vi "UHR-Fleezers Control (host) - Lorentz v4.vi"() -> ()   [LabVIEW 2014] (continued)
    n3458 = call-poly <vilib>:"Mean.vi"("X"=w4753) -> ("mean"=w4652:dbl)  [unwired: 1 out]
    "T2 X" <- w4652
    n3459 = Subtract(x=w4607, y=w4748) -> (x-y=w4747:dbl[])
    n3460 = Add(1:w4577, 2:w4581) -> (0:w4580:waveform(dbl))  [unwired: 1 in, 1 out]
    n3461 = Square(x=w4747) -> (x^2=w4746:dbl[])
    n3462 = Divide(x=w4580, y=2.0) -> (x/y=w4578:waveform(dbl))
    n3463 = Negate(x=w4753) -> (-x=w4619:dbl[])
    n3464 = call-poly <vilib>:"Mean.vi"("X"=w4746) -> ("mean"=w4745:dbl)  [unwired: 1 out]
    n3465 = Negate(x=w4652) -> (-x=w4651:dbl)
    n3466 = Square Root(x=w4745) -> (sqrt(x)=w4744:dbl)
    n3467 = Add(x=w4650, y=w4619) -> (x+y=w4754:dbl[])
    n3468 = Add(x=w4653, y=w4651) -> (x+y=w4772:dbl)
    n3469 = Multiply(x=10.0, y=w4744) -> (x*y=→"RMS (Ang)":dbl)
    n3470 = Divide(x=w4754, y=2.0) -> (x/y=w4622:dbl[])
    n3471 = Subtract(x=w4653, y=w4651) -> (x-y=→"Difference":dbl)
    n3472 = Build Array(w4581, w4577, w4578) -> (→"Force":waveform(dbl)[])
    n3473 = Select(t=w4619, s="Only check fixed trap T2", f=w4622) -> (s? t:f=→"Vec Mean of T1 T2":dbl[])
    n3474 = Divide(x=w4772, y=2.0) -> (x/y=w4563:dbl)
    "Mean" <- w4563
    n3475 = feedback-in #17("Trap Trig. Fl.") -> ()
    n3476 = feedback #17("Trap Trig. Fl.") -> (w4669:bool)
    n3477 = And(x=w4671, y=w4669) -> (x .and. y?=w4670:bool)
    n3478 = case "If have just turned off triggering" shown="True" w4670 {
      tunnel: w4574 -> [_ w4998]
      tunnel: w4665 -> [_ w4997]
      frame False {
      }
      frame True {
        w4996 = FALSE ("FPGA Trap Trig")
        n3479 = xnode "Read/Write Control"("FPGA VI Reference In"=w4998, "error in"=w4997, "FPGA Trap Trig"=w4996) -> ("FPGA VI Reference Out"=w4995:T50, "error out"=w4994:errorcluster)
        n3480 = xnode "Read/Write Control"("FPGA VI Reference In"=w4995, "error in"=w4994, "TTrig?"=w4996) -> ()  [unwired: 2 out]
        n3481 = local write "Initializing"(FALSE ("Initializing")) -> ()
        n3482 = local write "Triggered"(FALSE ("Triggered")) -> ()
        n3483 = local write "Waiting"(FALSE ("Waiting")) -> ()
      }
    }
    n3484 = Not(x=w4669) -> (.not. x?=w4682:bool)
    n3485 = And(x="Trap Trig. Fl.", y=w4682) -> (x .and. y?=w4679:bool)
    n3486 = Or(x=w4679, y="Reinitialize") -> (x .or. y?=w4668:bool)
    n3487 = feedback #18(w4675) -> (w4680:string)
    n3488 = Select(t=w4675, s=w4679, f=w4680) -> (s? t:f=w4674:string)
    n3489 = Select(t=w4675, s="Reinitialize", f=w4674) -> (s? t:f=w4673:string)
    n3490 = local read "Tether"() -> (w4756:bool)
    n3491 = feedback #19(0) -> (w4677:i32)
    n3492 = case "For determining if there is a tether still" shown="True" w4756 {
      tunnel: w4563 -> [_ w5107]
      frame False {
      }
      frame True {
        n3493 = Greater?(x="Lost Tether Alarm Threshold (pN)", y=w5107) -> (0:w5105:bool)
        n3494 = case shown="True" w5105 {
          frame False {
          }
          frame True {
            w5108 = FALSE ("Value (Signaling)")
            n3495 = flat-sequence {
              frame #0 {
                # "stop only if saving"
                n3496 = local read "Saving..."() -> (w5120:bool)
                n3497 = And(x=w5120, y="TA Cancel Save?") -> (x .and. y?=w5119:bool)
                n3498 = local write "Stop Saving"(w5119) -> ()
              }
              frame #1 {
                n3499 = case shown="True" "TA Green Off?" {
                  frame False {
                  }
                  frame True {
                    w5123 = FALSE ("Fl. Triggered...")
                    n3500 = local write "Fl. Triggered..."(w5123) -> ()
                    n3501 = property on="Green Laser ON" class="Bool (strict)"("Val(Sgnl)"=w5123) -> ()  [unwired: 2 in, 2 out]
                  }
                }
              }
            }
            n3502 = local read "Time tether formed"() -> (w5114:timestamp)
            n3503 = Get Date/Time In Seconds() -> (seconds since 1Jan1904=w5115:timestamp)
            n3504 = Subtract(x=w5115, y=w5114) -> (x-y=w5113:dbl)
            n3505 = Number To Decimal String(number=w5113) -> (decimal integer string=w5110:string)  [unwired: 1 out]
            n3506 = local read "Messages"() -> (w5117:string)
            n3507 = call <vilib>:"Beep.vi"() -> ()  [unwired: 3 in, 9 out]
            n3508 = Concatenate Strings("Lost tether (" ("Message to add"), w5110, " s)." ("string")) -> (w5112:string)
            n3509 = local write "Tether"(FALSE ("Tether")) -> ()
            n3510 = call "Update messages.vi"("Message to add"=w5112, "Old message string"=w5117) -> ("New message string"=w5116:string)
            n3511 = local write "Messages"(w5116) -> ()
            n3512 = property on="Fl. Triggered..." class="Bool (strict)"("Val(Sgnl)"=w5108) -> ()  [unwired: 2 in, 2 out]
            n3513 = local write "Dip for Protein"(w5108) -> ()
            n3514 = property on="Trap Pos. FB ON" class="Bool (strict)"("Val(Sgnl)"=w5108) -> ()  [unwired: 2 in, 2 out]
            n3515 = property on="Trap Trig. Fl." class="Bool (strict)"("Val(Sgnl)"=w5108) -> ()  [unwired: 2 in, 2 out]
          }
        }
      }
    }
    n3516 = case "For triggering actions based on the trap position (e.g., turning the excitation laser on if trap under feedback moves so far)" shown="True" "Trap Trig. Fl." {
      tunnel: w4479 -> [_ w5011]
      tunnel: w4673 -> [_ w5010]
      tunnel: ["" ("t") w5009] -> w4681
      tunnel: w4668 -> [_ w5008]
      tunnel: [0 ("t") w5007] -> w4678
      tunnel: w4677 -> [_ w5006]
      tunnel: w4574 -> [_ w5005]
      tunnel: w4665 -> [_ w5004]
      frame False {
      }
      frame True {
        n3517 = case shown="\"Wait for trigger\"" w5010 {
          tunnel: w5011 -> [w5028 _ _ w5076]
          tunnel: [w5025 w5057 "" ("t") w5079] -> w5009
          tunnel: w5008 -> [_ _ _ w5067]
          tunnel: [w5024 w5054 0 ("t") w5068] -> w5007
          tunnel: w5006 -> [_ w5056 _ w5074]
          tunnel: w5005 -> [w5013 w5051 _ w5070]
          tunnel: w5004 -> [w5012 w5050 _ w5069]
          frame "Wait for trigger" {
            n3518 = local read "Trap Trig. (FPGA)"() -> (w5016:bool)
            n3519 = Subtract(x=w5028, y="Mean T1 Position\nto compare (nm)") -> (x-y=w5021:dbl[])
            n3520 = call <vilib>:"Std Deviation and Variance.vi"("X"=w5021) -> ("mean"=→"mean":dbl, "standard deviation"=→"standard\ndeviation":dbl)  [unwired: 1 in, 1 out]
            n3521 = Array Max & Min(array=w5021) -> (max value=→"max value":dbl, min value=→"min value":dbl)  [unwired: 2 out]
            n3522 = Greater?(x=w5021, y="Threshold (nm)") -> (0:w5031:bool[])
            n3523 = case shown="True" w5016 {
              tunnel: w5013 -> [_ w5037]
              tunnel: w5012 -> [_ w5036]
              tunnel: [FALSE ("TTrig?") w5035] -> w5019
              frame False {
              }
              frame True {
                n3524 = xnode "Read/Write Control"("FPGA VI Reference In"=w5037, "error in"=w5036) -> ("TTrig?"=w5035:bool)  [unwired: 2 out]
              }
            }
            n3525 = Or Array Elements(Boolean array=w5031) -> (logical OR=w5018:bool)
            n3526 = Select(t=w5019, s=w5016, f=w5018) -> (s? t:f=w5017:bool)
            n3527 = Not(x=w5016) -> (.not. x?=w5015:bool)
            n3528 = And(x=w5017, y=w5015) -> (x .and. y?=w5014:bool)
            n3529 = Select(t="Triggered", s=w5017, f="Wait for trigger") -> (s? t:f=w5025:string)
            n3530 = case shown="True" w5017 {
              tunnel: [0 0] -> w5024
              tunnel: w5013 -> [_ w5042]
              tunnel: w5012 -> [_ w5041]
              frame False {
                "Waiting" <- TRUE ("Waiting")
              }
              frame True {
                n3531 = xnode "Read/Write Control"("FPGA VI Reference In"=w5042, "error in"=w5041, "TTrig?"=FALSE) -> ()  [unwired: 2 out]
                n3532 = local read "Messages"() -> (w5045:string)
                n3533 = call <vilib>:"Beep.vi"() -> ()  [unwired: 12 in]
                n3534 = call "Update messages.vi"("Message to add"="Unwinding trigger.", "Old message string"=w5045) -> ("New message string"=w5046:string)
                n3535 = local write "Messages"(w5046) -> ()
                n3536 = local write "Waiting"(FALSE ("Waiting")) -> ()
                "Triggered" <- TRUE ("Triggered")
              }
            }
            n3537 = case "Only need to turn on laser if host triggered" shown="True" w5014 {
              frame False {
              }
              frame True {
                n3538 = property on="Green Laser ON" class="Bool (strict)"("Val(Sgnl)"=TRUE ("Value (Signaling)")) -> ()  [unwired: 2 in, 2 out]
              }
            }
          }
          frame "Triggered" {
            n3539 = local read "Trap Trig. (FPGA)"() -> (w5053:bool)
            n3540 = Increment(x=w5056) -> (x+1=w5054:i32)
            n3541 = Greater Or Equal?(x=w5054, y="Fl. ON time (n)") -> (x >= y?=w5052:bool)
            n3542 = Select(t="Wait for trigger", s=w5052, f="Triggered" ("t")) -> (s? t:f=w5057:string)
            n3543 = And(x=w5052, y=w5053) -> (x .and. y?=w5049:bool)
            n3544 = case shown="True" w5049 {
              tunnel: w5051 -> [_ w5061]
              tunnel: w5050 -> [_ w5060]
              frame False {
              }
              frame True {
                n3545 = xnode "Read/Write Control"("FPGA VI Reference In"=w5061, "error in"=w5060, "FPGA Trap Trig"=TRUE) -> ()  [unwired: 2 out]
              }
            }
            n3546 = case shown="True" w5052 {
              frame False {
              }
              frame True {
                w5063 = FALSE ("Value (Signaling)")
                n3547 = local write "Triggered"(w5063) -> ()
                n3548 = local write "Waiting"(TRUE ("Waiting")) -> ()
                n3549 = property on="Green Laser ON" class="Bool (strict)"("Val(Sgnl)"=w5063) -> ()  [unwired: 2 in, 2 out]
              }
            }
          }
          frame "Do nothing" {
          }
          frame "Initialize", Default {
            n3550 = Increment(x=w5074) -> (x+1=w5078:i32)
            n3551 = Select(t=1, s=w5067, f=w5078) -> (s? t:f=w5068:i32)
            n3552 = feedback #20(w5076) -> (w5082:dbl[])
            n3553 = Build Array (concatenate)(w5076, w5082) -> (w5075:dbl[])
            n3554 = Greater Or Equal?(x=w5068, y="Wait to get offset (n)") -> (x >= y?=w5071:bool)
            n3555 = Select(t=w5076, s=w5067, f=w5075) -> (s? t:f=w5077:dbl[])
            n3556 = feedback-in #20(w5077) -> ()
            n3557 = call-poly <vilib>:"Mean.vi"("X"=w5077) -> ("mean"=w5072:dbl)  [unwired: 1 out]
            n3558 = local write "Mean T1 Position\nto compare (nm)"(w5072) -> ()
            n3559 = case shown="True" w5067 {
              tunnel: w5070 -> [_ w5088]
              tunnel: w5069 -> [_ w5087]
              frame False {
              }
              frame True {
                w5084 = FALSE ("FPGA Trap Trig")
                n3560 = xnode "Read/Write Control"("FPGA VI Reference In"=w5088, "error in"=w5087, "FPGA Trap Trig"=w5084) -> ("FPGA VI Reference Out"=w5086:T50, "error out"=w5085:errorcluster)
                n3561 = xnode "Read/Write Control"("FPGA VI Reference In"=w5086, "error in"=w5085, "TTrig?"=w5084) -> ()  [unwired: 2 out]
              }
            }
            n3562 = Select(t="Wait for trigger", s=w5071, f="Initialize") -> (s? t:f=w5079:string)
            n3563 = case shown="True" w5071 {
              tunnel: w5072 -> [_ w5091]
              tunnel: w5070 -> [_ w5100]
              tunnel: w5069 -> [_ w5099]
              frame False {
                n3564 = local write "Waiting"(FALSE ("Waiting")) -> ()
                "Initializing" <- TRUE ("Initializing")
              }
              frame True {
                n3565 = local read "Threshold (nm)"() -> (w5103:dbl)
                n3566 = local read "AOM X Cal (nm/MHz)"() -> (w5102:dbl)
                n3567 = Add(x=w5091, y=w5103) -> (x+y=w5104:dbl)
                n3568 = Divide(x=w5104, y=w5102) -> (x/y=w5101:dbl)
                n3569 = call "IR AOM freq to word.vi"("Frequency In (MHz)"=w5101) -> ("Frequency Word Out (double)"=w5098:dbl)
                n3570 = local write "Initializing"(FALSE ("Initializing")) -> ()
                n3571 = local write "Waiting"(TRUE ("Waiting")) -> ()
                n3572 = To Quad Integer(1:w5098) -> (0:w5097:i64)
                n3573 = xnode "Read/Write Control"("FPGA VI Reference In"=w5100, "error in"=w5099, "FPGA TTrig Thresh"=w5097) -> ("FPGA VI Reference Out"=w5094:T50, "error out"=w5093:errorcluster)
                n3574 = xnode "Read/Write Control"("FPGA VI Reference In"=w5094, "error in"=w5093, "FPGA Trap Trig"=TRUE) -> ()  [unwired: 2 out]
              }
            }
          }
        }
      }
    }
    n3575 = feedback-in #18(w4681) -> ()
    n3576 = feedback-in #19(w4678) -> ()
    n3577 = xnode ("Read/Write Control")("FPGA VI Reference In"=w4473, "error in"=w4764) -> ("FPGA VI Reference Out"=w4565:T50, "error out"=w4666:errorcluster, "AI2 Y Sum Set 1"=w4813:i16, "AI2 Y Sum Set 2"=w4812:i16, "AI1 X Set 1"=w4704:fxp<+/-,16,1>, "AI1 X Set 2"=w4703:fxp<+/-,16,1>, "Trap Pos FB Int Signal"=→"Trap Pos FB Int Signal":fxp<+/-,24,9>, "Trap Pos FB Int-Norm Signal"=→"Trap Pos FB Int-Norm Signal":fxp<+/-,16,1>, "Trap Pos FB Action"=w4697:i64, "Scanning"=→"AOD Scanning":bool, "Scan I"=→"AOD Scan I":u64, "Scanning MCL"=w4815:bool, "Scan I (MCL)"=→"MCL Scan I":u64, "Green FB Sum"=w4777:i16, "Trap Pos FB Action"=w4664:i64, "TTrig Fin Thresh"=w4660:i64, "Red FB Intensity"=w4647:i16, "Blue Intensity"=w4642:i16, "BD1 Frequency Out 1"=w4582:u64)
    "MCL Scanning" <- w4815
    "Trap Pos FB Action" <- w4697
    n3578 = Divide(x=w4647, y=3276.7) -> (x/y=w4646:dbl)
    "Red laser intensity (V)" <- w4646
    n3579 = Divide(x=w4642, y=3276.7) -> (x/y=w4641:dbl)
    "Blue laser intensity (V)" <- w4641
    n3580 = Divide(x=w4777, y=3276.7) -> (x/y=w4645:dbl)
    "Green laser intensity (V)" <- w4645
    n3581 = local read "FB Trig Integrate"() -> (w4658:u32)
    n3582 = Divide(x=w4664, y=w4658) -> (x/y=w4657:dbl)
    "TTrig Sig (Int)" <- w4657
    n3583 = Bundle(w4645, w4646, w4641) -> (→"Fluorescence laser intensities plot":cluster{dbl, dbl, dbl})  [unwired: 1 in]
    n3584 = Divide(x=w4660, y=w4658) -> (x/y=w4655:dbl)
    "TTrig Fin Thresh (Int)" <- w4655
    n3585 = local read "AOM X Cal (nm/MHz)"() -> (w4663:dbl)
    n3586 = local read "AI2 (V)"() -> (w4814:cluster{"Set 1":dbl, "Set 2":dbl})
    n3587 = Bundle By Name(cluster=w4814, "Set 1"=w4813, "Set 2"=w4812) -> (w4584:cluster{"Set 1":dbl, "Set 2":dbl})
    n3588 = Divide(x=w4697, y=327.67) -> (x/y=→"Action (%)":dbl)
    n3589 = case shown="True" "Semi Passive Mode" {
      tunnel: w4563 -> [_ w4881]
      frame False {
      }
      frame True {
        n3590 = local read "Target Force (pN)"() -> (w4879:dbl)
        n3591 = Less?(x="Jump Force (pN)", y=w4879) -> (x < y?=w4877:bool)
        n3592 = case shown="False" w4877 {
          tunnel: "Jump Force (pN)" -> [w4887 w4890]
          tunnel: w4881 -> [w4886 w4889]
          tunnel: [w4885 w4888] -> w4880
          frame False {
            n3593 = Less?(x=w4887, y=w4886) -> (x < y?=w4885:bool)
          }
          frame True {
            n3594 = Greater?(x=w4890, y=w4889) -> (0:w4888:bool)
          }
        }
        n3595 = case shown="False" w4880 {
          frame False {
            n3596 = local read "Trap Pos. FB ON"() -> (w4882:bool)
            n3597 = case shown="False" w4882 {
              frame False {
              }
              frame True {
                n3598 = property on="Trap Pos. FB ON" class="Bool (strict)"("Val(Sgnl)"=FALSE) -> ()  [unwired: 2 in, 2 out]
              }
            }
          }
          frame True {
            n3599 = property on="Trap Pos. FB ON" class="Bool (strict)"("Val(Sgnl)"=TRUE) -> ()  [unwired: 2 in, 2 out]
          }
        }
      }
    }
    n3600 = local read "Trap X (AI1)"() -> (w4717:T15)
    n3601 = call "IR AOM word double to freq.vi"("Frequency Word In (double)"=w4655) -> ("Frequency Out (MHz)"=w4654:dbl)
    n3602 = call "IR AOM word double to freq.vi"("Frequency Word In (double)"=w4657) -> ("Frequency Out (MHz)"=w4656:dbl)
    n3603 = Divide(x=w4584, y=3276.7) -> (x/y=w4810:cluster{"Set 1":dbl, "Set 2":dbl})
    n3604 = Multiply(x=w4656, y=w4663) -> (x*y=w4662:dbl)
    "TTrig Sig (nm)" <- w4662
    n3605 = Multiply(x=w4654, y=w4663) -> (x*y=w4661:dbl)
    "TTrig Fin Thresh (nm)" <- w4661
    n3606 = local write "AI2 (V)"(w4810) -> ()
    n3607 = Bundle(cluster=w4717, "Trap 1"=w4704, "Trap 2"=w4703) -> (→"Trap X (AI1)":T15)
    n3608 = local read "Trap Pos. FB ON"() -> (w4570:bool)
    n3609 = local read "Dynamic Force FB (ronen)"() -> (w4571:bool)
    n3610 = Bundle(w4662, w4661) -> (→"TTrig":cluster{dbl, dbl})  [unwired: 1 in]
    n3611 = Compound Arithmetic op=AND(w4571, "Real time Offset file correction for setpoint", w4570) -> (w4572:bool)
    n3612 = case shown="True" w4572 {
      tunnel: w4582 -> [_ _]
      tunnel: w4568 -> [_ w4909]
      tunnel: w4565 -> [_ w4892]
      frame False {
      }
      frame True {
        # "Changed by Ronen - real time update of set point\naccording to offset file"
        n3613 = local read "T1 calibration"() -> (w4904:T9)
        n3614 = local read "Offset file step size"() -> (w4911:dbl)
        n3615 = local read "Setpoint offset\ncorrection values"() -> (w4908:dbl[])
        n3616 = Multiply(x="Target Force (pN)", y=2.0) -> (x*y=w4905:dbl)
        n3617 = local read "Negate Diff?"() -> (w4893:bool)
        n3618 = Unbundle By Name(w4904) -> ("T1 alpha_x (nm/V)"=w4903:dbl, "T1 kappa_x (pN/nm)"=w4902:dbl)
        n3619 = Divide(x=w4909, y=w4911) -> (x/y=w4912:dbl)
        n3620 = To Long Integer(number=w4912) -> (32bit integer=w4910:i32)
        n3621 = Index Array(array=w4908, index=w4910) -> (element=w4895:dbl)
        n3622 = Multiply(x=w4903, y=w4902) -> (x*y=w4901:dbl)
        n3623 = Select(t=1, s=w4893, f=-1) -> (s? t:f=w4896:i32)
        n3624 = Divide(x=w4905, y=w4901) -> (x/y=w4900:dbl)
        n3625 = Multiply(x=w4896, y=w4895) -> (x*y=w4894:dbl)
        n3626 = Add(x=w4900, y=w4894) -> (x+y=w4899:dbl)
        n3627 = To Fixed-Point(number=w4899) -> (fixed-point=w4891:fxp<+/-,16,1>)  [unwired: 1 in]
        "Actual Setpoint" <- w4891
        n3628 = xnode "Read/Write Control"("FPGA VI Reference In"=w4892, "Trap Pos. FB SP"=w4891) -> ()  [unwired: 1 in, 2 out]
      }
    }
    n3629 = local read "All FB On/Off"() -> (w4583:bool)
    n3630 = case shown="True" w4583 {
      tunnel: w4584 -> [_ w4915]
      frame False {
      }
      frame True {
        n3631 = Divide(x=w4915, y=3276.7) -> (x/y=w4913:cluster{"Set 1":dbl, "Set 2":dbl})
        n3632 = Unbundle By Name(w4913) -> ("Set 1"=w4920:dbl, "Set 2"=w4919:dbl)
        n3633 = Greater?(x=w4920, y="Feedback Auto-Off threshold") -> (0:w4918:bool)
        n3634 = Greater?(x=w4919, y="Feedback Auto-Off threshold") -> (0:w4917:bool)
        n3635 = Or(x=w4918, y=w4917) -> (x .or. y?=w4916:bool)
        n3636 = case shown="True" w4916 {
          frame False {
          }
          frame True {
            n3637 = property on="All FB On/Off" class="Bool (strict)"("Val(Sgnl)"=FALSE) -> ()  [unwired: 2 in, 2 out]
          }
        }
      }
    }
    n3638 = flat-sequence "To save data" {
      tunnel: [w5618] -> w4833
      tunnel: [w5619] -> w4832
      tunnel: w4795 -> [w5612]
      tunnel: w4506 -> [w5616]
      tunnel: ["Save Calibration"] -> w4807
      tunnel: w4554 -> [w5615]
      tunnel: [w5608] -> w4804
      tunnel: [w5605] -> w4803
      tunnel: [w5602] -> w4802
      tunnel: w4794 -> [w5604]
      tunnel: w4533 -> [w5598]
      tunnel: [w5598] -> w4758
      tunnel: ["Start Saving"] -> w4738
      tunnel: [w5593] -> w4687
      tunnel: [w5592] -> w4686
      tunnel: [w5589] -> w4588
      tunnel: [w5585] -> w4576
      tunnel: w4833 -> [w5930]
      tunnel: w4832 -> [w5929]
      tunnel: w4555 -> [w5928]
      tunnel: w4807 -> [w5927]
      tunnel: w4804 -> [w5925]
      tunnel: w4803 -> [w5924]
      tunnel: w4802 -> [w5923]
      tunnel: w4529 -> [w5922]
      tunnel: w4550 -> [w5921]
      tunnel: w4758 -> [w5920]
      tunnel: w4738 -> [w5919]
      tunnel: w4595 -> [w5918]
      tunnel: w4637 -> [w5917]
      tunnel: w4687 -> [w5916]
      tunnel: w4686 -> [w5915]
      tunnel: w4685 -> [w5914]
      tunnel: w4478 -> [w5913]
      tunnel: w4544 -> [w5912]
      tunnel: w4588 -> [w5911]
      tunnel: w4576 -> [w5910]
      frame #0 {
        # "Changed by Ronen - we don't have a database so we disabled this"
        n3639 = Or(x="Save N Sets", y="Start Saving") -> (x .or. y?=w5599:bool)
        n3640 = To Double Precision Float(number=w5615) -> (double precision float=w5609:dbl)
        n3641 = Build Array(w5599, "Save Calibration", w5612, w5604, "Flow Cal") -> (w5614:bool[])
        n3642 = Compound Arithmetic op=OR("Save Calibration", w5612, w5599, w5604, "Flow Cal") -> (w5617:bool)
        n3643 = Boolean Array To Number(Boolean array=w5614) -> (number=w5611:u32)
        n3644 = feedback #21(FALSE ("Save APD Data\nwith Trap Data")) -> (w5594:bool)
        n3645 = feedback #22(refnum<k0> refnum) -> (w5620:refnum<file>)
        n3646 = feedback #23(FALSE ("Save APD Data\nwith Trap Data")) -> (w5603:bool)
        n3647 = feedback #24(0) -> (w5622:i32)
        n3648 = feedback #25() -> (w5610:u32)  [unwired: 1 out]
        n3649 = feedback #26(refnum<k0> refnum) -> (w5590:refnum<file>)
        n3650 = feedback #27(refnum<k0> refnum) -> (w5596:refnum<file>)
        n3651 = feedback #28(refnum<k0> refnum) -> (w5586:refnum<file>)
        n3652 = feedback #29(refnum<k0> refnum) -> (w5606:refnum<file>)
        n3653 = case shown="True" w5617 {
          tunnel: [w5631 1] -> w5618
          tunnel: w5622 -> [w5633 _]
          tunnel: [w5632 w5665] -> w5619
          tunnel: w5620 -> [w5632 _]
          tunnel: w5616 -> [_ w5683]
          tunnel: w5609 -> [_ w5681]
          tunnel: w5611 -> [_ w5684]
          tunnel: [w5630 w5664] -> w5608
          tunnel: w5610 -> [w5630 _]
          tunnel: [w5629 w5662] -> w5605
          tunnel: w5606 -> [w5629 _]
          tunnel: [w5628 w5661] -> w5602
          tunnel: w5603 -> [w5628 _]
          tunnel: "Start Saving" -> [_ w5659]
          tunnel: w5598 -> [_ w5658]
          tunnel: [w5627 w5651] -> w5592
          tunnel: w5596 -> [w5627 _]
          tunnel: [w5626 w5650] -> w5593
          tunnel: w5594 -> [w5626 _]
          tunnel: [w5625 w5636] -> w5589
          tunnel: w5590 -> [w5625 _]
          tunnel: [w5624 w5634] -> w5585
          tunnel: w5586 -> [w5624 _]
          frame False {
            n3654 = Increment(x=w5633) -> (x+1=w5631:i32)
          }
          frame True {
            w5635 = FALSE ("Start Saving")
            w5660 = 10.0  # File Version
            w5667 = FALSE ("prepend array or string size? (T)")
            w5666 = T38."big-endian, network order" ("byte order (0:big-endian, network order)")
            # "Ronen Changed the create file - changed data folder to c:\\Data"
            # "Save trap position\ndata"
            n3655 = Array Size(array=w5658) -> (size(s)=w5657:i32)
            n3656 = To Double Precision Float(number=w5657) -> (double precision float=w5656:dbl)
            n3657 = local read "BD 1 Frequency 1 (MHz)"() -> (w5680:dbl)
            n3658 = local read "BD 2 Frequency 1 (MHz)"() -> (w5679:dbl)
            n3659 = local read "BD 1 Frequency 2 (MHz)"() -> (w5678:dbl)
            n3660 = local read "BD 2 Frequency 2 (MHz)"() -> (w5677:dbl)
            n3661 = local read "BD 1 Frequency 3 (MHz)"() -> (w5676:dbl)
            n3662 = local read "BD 2 Frequency 3 (MHz)"() -> (w5675:dbl)
            n3663 = local write "Flow Cal"(w5635) -> ()
            n3664 = local write "Save Calibration"(w5635) -> ()
            n3665 = local write "Start Saving"(w5635) -> ()
            n3666 = Build Array("Save APD Data\nwith Trap Data", "Save Trap Pos. Data") -> (w5653:bool[])
            n3667 = Boolean Array To Number(Boolean array=w5653) -> (number=w5652:u32)
            n3668 = Build Array(w5680, w5679, w5678, w5677, w5676, w5675) -> (w5674:dbl[])
            n3669 = case shown="16" w5684 {
              tunnel: w5683 -> [w5784 w5811 w5827 w5865 w5902]
              tunnel: w5656 -> [w5789 w5818 w5847 w5884 w5907]
              tunnel: w5681 -> [w5788 w5817 w5846 w5883 w5906]
              tunnel: [w5785 w5813 w5838 w5875 w5903] -> w5672
              tunnel: [w5776 "Cal sets to save" w5828 w5866 w5889] -> w5664
              tunnel: w5674 -> [w5786 w5814 w5840 w5877 w5904]
              tunnel: "Save APD Data\nwith Trap Data" -> [w5783 w5800 w5824 w5863 w5901]
              tunnel: [w5783 w5798 w5824 w5863 w5901] -> w5661
              tunnel: w5660 -> [w5779 w5807 w5822 w5861 w5897]
              tunnel: w5659 -> [w5778 _ _ _ _]
              tunnel: [w5769 w5806 w5821 w5851 w5896] -> w5650
              tunnel: "Save Trap Pos. Data" -> [w5769 w5805 w5821 w5851 w5896]
              tunnel: w5652 -> [w5768 w5804 w5820 w5850 w5895]
              frame 1, Default {
                # "timeseries"
                n3670 = case shown="True" "Profile" {
                  tunnel: [w5792 w5796] -> w5773
                  tunnel: [w5792 w5795] -> w5772
                  tunnel: [w5792 w5794] -> w5771
                  tunnel: [w5792 w5793] -> w5770
                  frame False {
                    w5792 = 0.0 ("f")
                  }
                  frame True {
                    n3671 = local read "Current Position"() -> (w5797:cluster{dbl, dbl, dbl})
                    n3672 = local read "Y change (mm)"() -> (w5793:dbl)
                    n3673 = Unbundle(w5797) -> (w5796:dbl, w5795:dbl, w5794:dbl)
                  }
                }
                n3674 = local read "Save ave N"() -> (w5791:dbl)
                n3675 = Multiply(x=w5791, y=w5784) -> (x*y=w5790:dbl)
                n3676 = To Double Precision Float(number=w5768) -> (double precision float=w5782:dbl)
                n3677 = Build Array(w5779, w5784, w5790, w5789, w5788, 0.0 ("f")) -> (w5787:dbl[])
                n3678 = Build Array(w5782, w5773, w5772, w5771, w5770) -> (w5780:dbl[])
                n3679 = Select(t=u32 4000000000, s=w5778, f="N sets to save") -> (s? t:f=w5776:u32)
                n3680 = Build Array (concatenate)(w5787, w5786, w5780) -> (w5785:dbl[])
              }
              frame 2 {
                w5809 = 0.0 ("f")
                w5799 = FALSE ("Save APD Data\nwith Trap Data")
                # "For diagnostics save trap position\ndata during cal"
                # "calibration"
                n3681 = Boolean To (0,1)(Boolean=w5799) -> (0, 1=w5803:i16)
                n3682 = Select(t=w5800, s="Save trap pos with cal", f=w5799) -> (s? t:f=w5798:bool)
                n3683 = Select(t=w5805, s="Save trap pos with cal", f=w5799) -> (s? t:f=w5806:bool)
                n3684 = Select(t=w5804, s="Save trap pos with cal", f=w5803) -> (s? t:f=w5802:u32)
                n3685 = To Double Precision Float(number=w5802) -> (double precision float=w5810:dbl)
                n3686 = Build Array(w5807, w5811, w5811, w5818, w5817, 1.0 ("t")) -> (w5815:dbl[])
                n3687 = Build Array(w5810, w5809, w5809, w5809, w5809) -> (w5808:dbl[])
                n3688 = Build Array (concatenate)(w5815, w5814, w5808) -> (w5813:dbl[])
                "Calibrating Trap..." <- TRUE ("Calibrating...")
              }
              frame 4 {
                w5825 = 0.0 ("f")
                # "scan dir (x/y = 0/1)"
                # "cycles/step"
                # "n scans (f/b)"
                # "steps"
                # "freq. range"
                # "AOD raster scan"
                n3689 = local read "Number of F/B Scans (AOD)"() -> (w5832:u16)
                n3690 = local read "Cycles/step (AOD)"() -> (w5834:u64)
                n3691 = local read "Scan Range (MHz)"() -> (w5837:dbl)
                n3692 = local read "Scan steps (AOD)"() -> (w5836:u64)
                n3693 = local read "Scan BD"() -> (w5844:bool)
                n3694 = local read "Save ave N"() -> (w5849:dbl)
                n3695 = Boolean To (0,1)(Boolean=w5844) -> (0, 1=w5843:i16)
                n3696 = To Double Precision Float(number=w5832) -> (double precision float=w5831:dbl)
                n3697 = To Double Precision Float(number=w5836) -> (double precision float=w5835:dbl)
                n3698 = To Double Precision Float(number=w5834) -> (double precision float=w5833:dbl)
                n3699 = To Double Precision Float(number=w5843) -> (double precision float=w5842:dbl)
                n3700 = Multiply(x=w5849, y=w5827) -> (x*y=w5848:dbl)
                n3701 = To Double Precision Float(number=w5820) -> (double precision float=w5826:dbl)
                n3702 = Build Array(w5826, w5825, w5825, w5825, w5825) -> (w5823:dbl[])
                n3703 = local read "N sets should be saved"() -> (w5829:dbl)
                n3704 = Build Array(w5842, w5837, w5835, w5833, w5831) -> (w5839:dbl[])
                n3705 = Build Array(w5822, w5827, w5848, w5847, w5846, 2.0 ("t")) -> (w5841:dbl[])
                n3706 = Round Toward +Infinity(x=w5829) -> (ceil(x): smallest int >= x=w5830:dbl)
                n3707 = Build Array (concatenate)(w5841, w5840, w5823, w5839) -> (w5838:dbl[])
                n3708 = To Unsigned Long Integer(number=w5830) -> (unsigned 32bit integer=w5828:u32)
              }
              frame 8 {
                w5858 = 0.0 ("f")
                # "MCL raster scan"
                n3709 = local read "Number of scans (MCL)"() -> (w5853:u64)
                n3710 = local read "2D or 1D Scan"() -> (w5855:bool)
                n3711 = local read "Scan lines (y)"() -> (w5852:u64)
                n3712 = local read "Scan Range (V)\n(of steps)"() -> (w5874:dbl)
                n3713 = local read "Fast Scan Dir"() -> (w5881:bool)
                n3714 = local read "Cycles/step (MCL)"() -> (w5871:u64)
                n3715 = local read "Scan steps (MCL)"() -> (w5873:u64)
                n3716 = Select(t=w5852, s=w5855, f=w5853) -> (s? t:f=w5854:u64)
                n3717 = Boolean To (0,1)(Boolean=w5855) -> (0, 1=w5857:i16)
                n3718 = local read "Save ave N"() -> (w5886:dbl)
                n3719 = local read "Initial X"() -> (w5860:dbl)
                n3720 = local read "Initial Y"() -> (w5859:dbl)
                n3721 = To Double Precision Float(number=w5857) -> (double precision float=w5856:dbl)
                n3722 = Boolean To (0,1)(Boolean=w5881) -> (0, 1=w5880:i16)
                n3723 = To Double Precision Float(number=w5854) -> (double precision float=w5869:dbl)
                n3724 = To Double Precision Float(number=w5873) -> (double precision float=w5872:dbl)
                n3725 = To Double Precision Float(number=w5871) -> (double precision float=w5870:dbl)
                n3726 = To Double Precision Float(number=w5880) -> (double precision float=w5879:dbl)
                n3727 = Multiply(x=w5886, y=w5865) -> (x*y=w5885:dbl)
                n3728 = To Double Precision Float(number=w5850) -> (double precision float=w5864:dbl)
                n3729 = local read "N sets should be saved (MCL)"() -> (w5867:dbl)
                n3730 = Build Array(w5864, w5856, w5858, w5858, w5858) -> (w5862:dbl[])
                n3731 = Build Array(w5879, w5874, w5872, w5870, w5869, w5860, w5859) -> (w5876:dbl[])
                n3732 = Build Array(w5861, w5865, w5885, w5884, w5883, 3.0 ("t")) -> (w5878:dbl[])
                n3733 = Round Toward +Infinity(x=w5867) -> (ceil(x): smallest int >= x=w5868:dbl)
                n3734 = Build Array (concatenate)(w5878, w5877, w5862, w5876) -> (w5875:dbl[])
                n3735 = To Unsigned Long Integer(number=w5868) -> (unsigned 32bit integer=w5866:u32)
              }
              frame 16 {
                w5888 = 0.0
                # "Flow calibration - added by Ronen: Number\nof saved sets is distance (1 mm) divided by \nspeed +1.5 spare second divided by the time of\nset measurement, 0.2 sec for 2 set interlace"
                # "timeseries"
                n3736 = local read "Save ave N"() -> (w5909:dbl)
                n3737 = Reciprocal(x=0.0) -> (1/x=w5894:dbl)
                n3738 = Add(x=w5894, y=1.5) -> (x+y=w5892:dbl)
                n3739 = Multiply(x=w5909, y=w5902) -> (x*y=w5908:dbl)
                n3740 = Divide(x=w5892, y=0.2) -> (x/y=w5890:dbl)
                n3741 = To Double Precision Float(number=w5895) -> (double precision float=w5900:dbl)
                n3742 = To Unsigned Long Integer(number=w5890) -> (unsigned 32bit integer=w5889:u32)
                n3743 = Build Array(w5897, w5902, w5908, w5907, w5906, 4.0 ("f")) -> (w5905:dbl[])
                n3744 = Build Array(w5900, w5888, w5888, w5888, w5888) -> (w5898:dbl[])
                n3745 = Build Array (concatenate)(w5905, w5904, w5898) -> (w5903:dbl[])
              }
            }
            n3746 = local read "Index"() -> (w5689:dbl)
            n3747 = call "Create new save file.vi"("Insert"="", "Ext"=".dat", "Index In"=w5689) -> ("Path Out"=w5638:path, "Index Out"=w5663:dbl)
            n3748 = local write "Save file name"(w5638) -> ()
            n3749 = local write "Index"(w5663) -> ()
            n3750 = local write "Save index"(w5663) -> ()
            n3751 = case shown="True" "Save Event Log?" {
              tunnel: w5638 -> [_ w5703]
              tunnel: [refnum<k0> refnum w5702] -> w5636
              frame False {
              }
              frame True {
                (unwired) FALSE ("prepend array or string size? (T)")
                n3752 = Path To String(path=w5703) -> (string=w5714:string)
                n3753 = String Length(string=w5714) -> (length=w5713:i32)
                n3754 = Subtract(x=w5713, y=4) -> (x-y=w5711:i32)
                n3755 = String Subset(string=w5714, length (rest)=w5711) -> (substring=w5710:string)  [unwired: 1 out]
                n3756 = Concatenate Strings(w5710, "_log.txt" ("string")) -> (w5708:string)
                n3757 = String To Path(string=w5708) -> (path=w5704:path)
                n3758 = Open/Create/Replace File(file path (use dialog)=w5704, operation (0:open)=T39."create", access (0:read/write)=enum16{"read/write", "read-only", "write-only"}."write-only") -> (refnum out=w5705:refnum<file>)  [unwired: 1 in, 4 out]
                n3759 = Deny Access(7:w5705) -> (3:w5702:refnum<file>)  [unwired: 1 in, 2 out]
                n3760 = call "write to event log.vi"("log file ref"=w5702, "time"=0.0, "input string"="start log") -> ()  [unwired: 8 in]
              }
            }
            "log file ref" <- w5636
            n3761 = Array Size(array=w5672) -> (size(s)=w5673:i32)
            n3762 = Open/Create/Replace File(file path (use dialog)=w5638, operation (0:open)=T39."create", access (0:read/write)=enum16{"read/write", "read-only", "write-only"}."write-only") -> (refnum out=w5686:refnum<file>)  [unwired: 1 in, 4 out]
            n3763 = local write "Saving..."(TRUE ("Saving...")) -> ()
            n3764 = To Double Precision Float(number=w5673) -> (double precision float=w5671:dbl)
            n3765 = String Length(string="Comment (data description)") -> (length=w5670:i32)
            n3766 = To Double Precision Float(number=w5670) -> (double precision float=w5669:dbl)
            n3767 = Deny Access(7:w5686) -> (3:w5685:refnum<file>)  [unwired: 1 in, 2 out]
            n3768 = Build Array (concatenate)(w5671, w5672, w5669) -> (w5648:dbl[])
            n3769 = case "If fluorescence data to be saved" shown="True" w5661 {
              tunnel: w5638 -> [_ w5767]
              tunnel: [w5737 w5750] -> w5662
              tunnel: [w5737 w5738] -> w5634
              frame False {
                w5737 = refnum<k0> refnum
              }
              frame True {
                w5749 = 0.0
                w5742 = T39."create" ("operation (0:open)")
                w5743 = enum16{"read/write", "read-only", "write-only"}."write-only" ("access (0:read/write)")
                n3770 = local read "APD Integration Time (s)"() -> (w5755:dbl)
                n3771 = local read "N APD Samp/step"() -> (w5748:dbl)
                n3772 = local read "Number of APDs"() -> (w5747:u8)
                n3773 = Path To String(path=w5767) -> (string=w5766:string)
                n3774 = String Length(string=w5766) -> (length=w5765:i32)
                n3775 = Subtract(x=w5765, y=4) -> (x-y=w5763:i32)
                n3776 = String Subset(string=w5766, length (rest)=w5763) -> (substring=w5746:string)  [unwired: 1 out]
                n3777 = Build Array(w5755, w5748, w5747, w5749, w5749, w5749, w5749, w5749) -> (w5752:dbl[])
                n3778 = Concatenate Strings(w5746, "_green.dat") -> (w5744:string)
                n3779 = Concatenate Strings(w5746, "_fl.dat" ("string")) -> (w5761:string)
                n3780 = Array Size(array=w5752) -> (size(s)=w5754:i32)
                n3781 = String To Path(string=w5761) -> (path=w5759:path)
                n3782 = Open/Create/Replace File(file path (use dialog)=w5759, operation (0:open)=w5742, access (0:read/write)=w5743) -> (refnum out=w5760:refnum<file>)  [unwired: 1 in, 4 out]
                n3783 = Deny Access(7:w5760) -> (3:w5756:refnum<file>)  [unwired: 1 in, 2 out]
                n3784 = String To Path(string=w5744) -> (path=w5741:path)
                n3785 = To Double Precision Float(number=w5754) -> (double precision float=w5753:dbl)
                n3786 = Build Array (concatenate)(w5753, w5752) -> (w5751:dbl[])
                n3787 = Write to Binary File(file (use dialog)=w5756, data=w5751, 5:FALSE ("prepend array or string size? (T)"), 9:T38."big-endian, network order" ("byte order (0:big-endian, network order)")) -> (refnum out=w5750:refnum<file>)  [unwired: 1 in, 3 out]
                n3788 = Open/Create/Replace File(file path (use dialog)=w5741, operation (0:open)=w5742, access (0:read/write)=w5743) -> (refnum out=w5739:refnum<file>, error out=w5740:errorcluster)  [unwired: 3 in, 1 out]
                n3789 = Deny Access(4:w5740, 7:w5739) -> (3:w5738:refnum<file>)  [unwired: 1 in, 1 out]
              }
            }
            n3790 = case shown="True" w5650 {
              tunnel: w5638 -> [_ w5722]
              tunnel: [refnum<k0> refnum w5721] -> w5651
              frame False {
              }
              frame True {
                w5717 = 0.0 ("element")
                n3791 = Path To String(path=w5722) -> (string=w5736:string)
                n3792 = Build Array(w5717, w5717, w5717, w5717, w5717, w5717, w5717, w5717) -> (w5718:dbl[])
                n3793 = String Length(string=w5736) -> (length=w5735:i32)
                n3794 = Subtract(x=w5735, y=4) -> (x-y=w5733:i32)
                n3795 = Array Size(array=w5718) -> (size(s)=w5720:i32)
                n3796 = String Subset(string=w5736, length (rest)=w5733) -> (substring=w5732:string)  [unwired: 1 out]
                n3797 = To Double Precision Float(number=w5720) -> (double precision float=w5719:dbl)
                n3798 = Concatenate Strings(w5732, "_pos.dat" ("string")) -> (w5730:string)
                n3799 = Build Array (concatenate)(w5719, w5718) -> (w5716:dbl[])
                n3800 = String To Path(string=w5730) -> (path=w5726:path)
                n3801 = Open/Create/Replace File(file path (use dialog)=w5726, operation (0:open)=T39."create", access (0:read/write)=enum16{"read/write", "read-only", "write-only"}."write-only") -> (refnum out=w5727:refnum<file>)  [unwired: 1 in, 4 out]
                n3802 = Deny Access(7:w5727) -> (3:w5723:refnum<file>)  [unwired: 1 in, 2 out]
                n3803 = Write to Binary File(file (use dialog)=w5723, data=w5716, 5:FALSE ("prepend array or string size? (T)"), 9:T38."big-endian, network order" ("byte order (0:big-endian, network order)")) -> (refnum out=w5721:refnum<file>)  [unwired: 1 in, 3 out]
              }
            }
            n3804 = Write to Binary File(file (use dialog)=w5685, data=w5648, 5:w5667, 9:w5666) -> (refnum out=w5668:refnum<file>)  [unwired: 1 in, 3 out]
            n3805 = Write to Binary File(file (use dialog)=w5668, data="Comment (data description)", 5:w5667, 9:w5666) -> (refnum out=w5665:refnum<file>)  [unwired: 1 in, 3 out]
            n3806 = local read "connection reference"() -> (w5649:T25)
            n3807 = Bundle("Comment (data description)"="Comment (data description)", "Channel 1 Buffer"="Channel 1 Buffer", "Channel 2 Buffer"="Channel 2 Buffer", "Channel 3 Buffer"="Channel 3 Buffer", "Title"="Title", "DNA Construct"="DNA Construct", "Bead diameter"="Bead diameter", "Name"="Name") -> (w5639:T73)  [unwired: 1 in]
            n3808 = disable-structure shown="Disabled" {
              disable-tunnel: w5649 -> [w5697 _]
              disable-tunnel: w5648 -> [w5695 _]
              disable-tunnel: w5639 -> [w5694 _]
              disable-tunnel: w5638 -> [w5693 _]
              frame Disabled {
                n3809 = call "MattFileCreator-v9.vi"("Comments"=w5694, "Input Array"=w5695, "File path"=w5693, "table"="labview", "connection reference"=w5697) -> ("connection reference out"=w5696:T25)  [unwired: 5 in, 1 out]
                n3810 = local write "connection reference"(w5696) -> ()
              }
              frame Enabled {
              }
            }
          }
        }
        n3811 = feedback-in #21(w5593) -> ()
        n3812 = feedback-in #22(w5619) -> ()
        n3813 = feedback-in #23(w5602) -> ()
        n3814 = feedback-in #24(w5618) -> ()
        n3815 = feedback-in #25(w5608) -> ()
        n3816 = feedback-in #26(w5589) -> ()
        n3817 = feedback-in #27(w5592) -> ()
        n3818 = feedback-in #28(w5585) -> ()
        n3819 = feedback-in #29(w5605) -> ()
      }
      frame #1 {
        n3820 = local read "Saving..."() -> (w5926:bool)
        n3821 = case shown="True" w5926 {
          tunnel: w5930 -> [_ w5944]
          tunnel: w5929 -> [_ w5958]
          tunnel: w5928 -> [_ w5954]
          tunnel: w5927 -> [_ w5953]
          tunnel: w5925 -> [_ w5952]
          tunnel: w5924 -> [_ w5947]
          tunnel: w5923 -> [_ w5946]
          tunnel: w5922 -> [_ w5945]
          tunnel: w5921 -> [_ w5943]
          tunnel: w5920 -> [_ w5941]
          tunnel: w5919 -> [_ w5940]
          tunnel: w5918 -> [_ w5939]
          tunnel: w5917 -> [_ w5938]
          tunnel: w5916 -> [_ w5937]
          tunnel: w5915 -> [_ w5936]
          tunnel: w5914 -> [_ w5935]
          tunnel: w5913 -> [_ w5934]
          tunnel: w5912 -> [_ w5933]
          tunnel: w5911 -> [_ w5932]
          tunnel: w5910 -> [_ w5931]
          frame False {
          }
          frame True {
            n3822 = Multiply(x=w5944, y=w5943) -> (x*y=→"Time (s)":dbl)
            n3823 = Less Or Equal?(x=w5944, y=w5952) -> (x <= y?=w5956:bool)
            n3824 = Compound Arithmetic op=OR("Stop Saving", "Abort save 2") -> (w5948:bool)
            n3825 = Not(x=w5948) -> (.not. x?=w5957:bool)
            n3826 = And(x=w5956, y=w5957) -> (x .and. y?=w5955:bool)
            n3827 = case shown="True" w5955 {
              tunnel: w5958 -> [w5968 w6069]
              tunnel: [0.0 w6072] -> w5951
              tunnel: w5944 -> [_ w6070]
              tunnel: w5952 -> [_ w6071]
              tunnel: w5954 -> [_ w6066]
              tunnel: w5953 -> [_ _]
              tunnel: w5947 -> [w5966 w6059]
              tunnel: w5946 -> [w5965 w6060]
              tunnel: w5945 -> [_ w6058]
              tunnel: w5941 -> [_ w6057]
              tunnel: w5940 -> [_ w5975]
              tunnel: w5939 -> [_ w6050]
              tunnel: w5938 -> [_ w5997]
              tunnel: w5937 -> [w5962 w6014]
              tunnel: w5936 -> [w5963 w6013]
              tunnel: w5935 -> [_ w6010]
              tunnel: w5934 -> [_ w6008]
              tunnel: w5933 -> [_ w5974]
              tunnel: w5932 -> [w5961 _]
              tunnel: w5931 -> [w5959 w5973]
              frame False {
                w5964 = FALSE
                n3828 = Close File(refnum=w5968) -> ()  [unwired: 1 in, 2 out]
                n3829 = case shown="True" w5965 {
                  tunnel: w5966 -> [_ w5972]
                  tunnel: w5959 -> [_ w5971]
                  frame False {
                  }
                  frame True {
                    n3830 = Close File(refnum=w5972) -> ()  [unwired: 1 in, 2 out]
                    n3831 = Close File(refnum=w5971) -> ()  [unwired: 1 in, 2 out]
                  }
                }
                n3832 = case shown="True" w5962 {
                  tunnel: w5963 -> [_ w5970]
                  frame False {
                  }
                  frame True {
                    n3833 = Close File(refnum=w5970) -> ()  [unwired: 1 in, 2 out]
                  }
                }
                n3834 = local read "Save Event Log?"() -> (w5960:bool)
                n3835 = case shown="True" w5960 {
                  tunnel: w5961 -> [_ w5969]
                  frame False {
                  }
                  frame True {
                    n3836 = Close File(refnum=w5969) -> ()  [unwired: 1 in, 2 out]
                  }
                }
                n3837 = local write "Raster Scanning..."(w5964) -> ()
                n3838 = local write "Calibrating Trap..."(w5964) -> ()
                n3839 = call <vilib>:"Beep.vi"() -> ()  [unwired: 3 in, 9 out]
                n3840 = local write "Stop Saving"(w5964) -> ()
                "Saving..." <- w5964
              }
              frame True {
                n3841 = local read "Calibrating Trap..."() -> (w6061:bool)
                n3842 = case "Write fl. data" shown="True" w6060 {
                  tunnel: w6059 -> [_ w6102]
                  tunnel: w6058 -> [_ w6101]
                  tunnel: w5973 -> [_ w6095]
                  frame False {
                  }
                  frame True {
                    w6094 = FALSE ("prepend array or string size? (T)")
                    w6096 = T38."big-endian, network order" ("byte order (0:big-endian, network order)")
                    n3843 = property on="Green Laser ON" class="Bool (strict)"() -> ("Value"=w6100:bool)  [unwired: 2 in, 2 out]
                    n3844 = property on="Green Intensity % (FB OFF)" class="DigNum (strict)"() -> ("Value"=w6099:dbl)  [unwired: 2 in, 2 out]
                    n3845 = Boolean To (0,1)(Boolean=w6100) -> (0, 1=w6098:i16)
                    n3846 = Multiply(x=w6098, y=w6099) -> (x*y=w6097:dbl)
                    n3847 = Write to Binary File(file (use dialog)=w6102, data=w6101, 5:w6094, 9:w6096) -> ()  [unwired: 1 in, 4 out]
                    n3848 = Write to Binary File(file (use dialog)=w6095, data=w6097, 5:w6094, 9:w6096) -> ()  [unwired: 2 in, 3 out]
                  }
                }
                n3849 = Greater?(x="Save ave N", y=1.0) -> (0:w6064:bool)
                n3850 = Not(x=w6061) -> (.not. x?=w6063:bool)
                n3851 = And(x=w6063, y=w6064) -> (x .and. y?=w6011:bool)
                n3852 = case shown="True" w6011 {
                  tunnel: w6010 -> [w6075 w6086]
                  tunnel: [w6075 w6078] -> w6009
                  tunnel: "Save ave N" -> [_ w6079]
                  frame False {
                  }
                  frame True {
                    w6076 = 2 ("dimension size")
                    n3853 = Array Size(array=w6086) -> (size(s)=w6080:i32)
                    n3854 = Divide(x=w6080, y=w6076) -> (x/y=w6084:dbl)
                    n3855 = Reshape Array(w6086, w6084, w6076) -> (w6085:u64[][])
                    n3856 = Transpose 2D Array(2D array=w6085) -> (transposed array=w6083:u64[][])
                    n3857 = for {
                      tunnel: w6083 -> [w6088] mode=indexing
                      tunnel: [w6087] -> w6077 mode=indexing
                      tunnel: w6079 -> [w6089]
                      workers-P: _ -> [_]
                      n3858 = call "downsample 1D array - U64.vi"("Ave N"=w6089, "Array In"=w6088) -> ("Array Out"=w6087:u64[])  [unwired: 1 in]
                    }
                    n3859 = Transpose 2D Array(2D array=w6077) -> (transposed array=w6082:u64[][])
                    n3860 = Divide(x=w6080, y=w6079) -> (x/y=w6081:dbl)
                    n3861 = Reshape Array(w6082, w6081) -> (w6078:u64[])
                  }
                }
                n3862 = case shown="True" w6011 {
                  tunnel: w6066 -> [w6103 w6115]
                  tunnel: [w6103 w6107] -> w6062
                  tunnel: "Save ave N" -> [_ w6108]
                  tunnel: w6057 -> [_ w6106]
                  frame False {
                  }
                  frame True {
                    n3863 = Array Size(array=w6115) -> (size(s)=w6109:i32)
                    n3864 = Array Size(array=w6106) -> (size(s)=w6105:i32)
                    n3865 = Divide(x=w6109, y=w6105) -> (x/y=w6113:dbl)
                    n3866 = Reshape Array(w6115, w6113, w6105) -> (w6114:i16[][])
                    n3867 = Transpose 2D Array(2D array=w6114) -> (transposed array=w6112:i16[][])
                    n3868 = for {
                      tunnel: w6112 -> [w6118] mode=indexing
                      tunnel: [w6117] -> w6104 mode=indexing
                      tunnel: w6108 -> [w6116]
                      workers-P: _ -> [_]
                      n3869 = call "downsample 1D array - I16 to F32.vi"("Ave N"=w6116, "Array In"=w6118) -> ("Array Out"=w6117:sgl[])  [unwired: 1 in]
                    }
                    n3870 = Transpose 2D Array(2D array=w6104) -> (transposed array=w6111:sgl[][])
                    n3871 = Divide(x=w6109, y=w6108) -> (x/y=w6110:dbl)
                    n3872 = Reshape Array(w6111, w6110) -> (w6107:sgl[])
                  }
                }
                n3873 = Index Array(array=w5997, index=2) -> (element=w5998:waveform(dbl))
                n3874 = Index Array(array=w5997, index=1) -> (element=w6031:waveform(dbl))
                n3875 = Index Array(array=w5997, index=0) -> (element=w6033:waveform(dbl))
                n3876 = Unbundle By Name(w5998) -> ("Y"=w6000:dbl[])
                n3877 = Unbundle By Name(w6031) -> ("Y"=w6035:dbl[])
                n3878 = Unbundle By Name(w6033) -> ("Y"=w6043:dbl[])
                n3879 = case "Write trap pos. data" shown="True" w6014 {
                  tunnel: w6013 -> [_ w6091]
                  tunnel: w6009 -> [_ w6090]
                  frame False {
                  }
                  frame True {
                    n3880 = Write to Binary File(file (use dialog)=w6091, data=w6090, 5:FALSE ("prepend array or string size? (T)"), 9:T38."big-endian, network order" ("byte order (0:big-endian, network order)")) -> ()  [unwired: 1 in, 4 out]
                  }
                }
                n3881 = Write to Binary File(file (use dialog)=w6069, data=w6062, 5:FALSE ("prepend array or string size? (T)"), 9:T38."big-endian, network order" ("byte order (0:big-endian, network order)")) -> ()  [unwired: 1 in, 4 out]
                n3882 = feedback #30(w6000) -> (w6001:dbl[])
                n3883 = Build Array (concatenate)(w6001, w6000) -> (w5996:dbl[])
                n3884 = Select(t=w6000, s=w5975, f=w5996) -> (s? t:f=w5986:dbl[])
                n3885 = feedback-in #30(w5986) -> ()
                n3886 = feedback #31(w6035) -> (w6037:dbl[])
                n3887 = Build Array (concatenate)(w6037, w6035) -> (w6036:dbl[])
                n3888 = Select(t=w6035, s=w5975, f=w6036) -> (s? t:f=w6025:dbl[])
                n3889 = feedback-in #31(w6025) -> ()
                n3890 = feedback #32(w6043) -> (w6056:dbl[])
                n3891 = Build Array (concatenate)(w6056, w6043) -> (w6055:dbl[])
                n3892 = Select(t=w6043, s=w5975, f=w6055) -> (s? t:f=w6030:dbl[])
                n3893 = feedback-in #32(w6030) -> ()
                n3894 = Divide(x=w6070, y=w6071) -> (x/y=w6073:dbl)
                n3895 = Multiply(x=w6073, y=100.0) -> (x*y=w6072:dbl)
                n3896 = Build Array(w6030, w6025, w5986) -> (→"Saved APD":dbl[][])
                n3897 = Array Size(array=w6030) -> (size(s)=w6048:i32)
                n3898 = Unbundle By Name(w6050) -> ("Y"=w6054:dbl[])
                n3899 = Subtract(x=w6048, y="N pts to average") -> (x-y=w5983:i32)
                n3900 = Multiply(x="N pts to average", y=u16 2) -> (x*y=w6026:u16)
                n3901 = Subtract(x=w6048, y=w6026) -> (x-y=w5984:i32)
                n3902 = feedback #33(w6054) -> (w6053:dbl[])
                n3903 = Build Array (concatenate)(w6053, w6054) -> (w6052:dbl[])
                n3904 = Select(t=w6054, s=w5975, f=w6052) -> (s? t:f=w6051:dbl[])
                "Trap Delta Graph" <- w6051
                n3905 = feedback-in #33(w6051) -> ()
                n3906 = Array Subset(array=w6030, index=w5983, length="N pts to average") -> (w6047:dbl[])
